vi "Test_PublishDblX_ObserveDblX_ValueReceived.vi"(8 "error in (no error)":errorcluster, 11 "TestCase in":refnum<class "TestModelPublishAndObserve.lvclass">) -> (0 "error out":errorcluster, 3 "TestCase out":refnum<class "TestModelPublishAndObserve.lvclass">)   [LabVIEW 2020, in "TestModelPublishAndObserve.lvclass"]
uses:
  TestModelPublishAndObserve.lvclass
  TestModelPublishAndObserve.lvclass/TestModelPublishAndObserve.ctl
  24bf8875-c008-4f22-9bfa-88e42476d167.vi
  Source/IModel/IModel/IModel.lvclass
  Doubles/RootModelPublishesDoubleFloatX/RootModelPublishesDoubleFloatX.lvclass
  C:/Git/mva-core/Source/RootModel/RootModel/RootModel.lvclass
  C:/Git/mva-core/Source/IModel/IModel/IModel.lvclass
  C:/Git/mva-core/Source/IObserver/IObserver/IObserver.lvclass
  C:/Program Files (x86)/National Instruments/LabVIEW 2020/vi.lib/ActorFramework/Actor/Actor.lvclass
  C:/Git/mva-core/Test/Doubles/RootModelPublishesDoubleFloatX/RootModelPublishesDoubleFloatX.lvclass
  <vilib>/ActorFramework/Actor/Actor.lvclass
  Source/Mediator/Mediator/Mediator.lvclass
  Doubles/ModelSubscribesToDoubleFloatX/ModelSubscribesToDoubleFloatX.lvclass
  <vilib>/ActorFramework/Stop Msg/Stop Msg.lvclass
  C:/Git/mva-core/Test/Doubles/ModelSubscribesToDoubleFloatX/ModelSubscribesToDoubleFloatX.lvclass
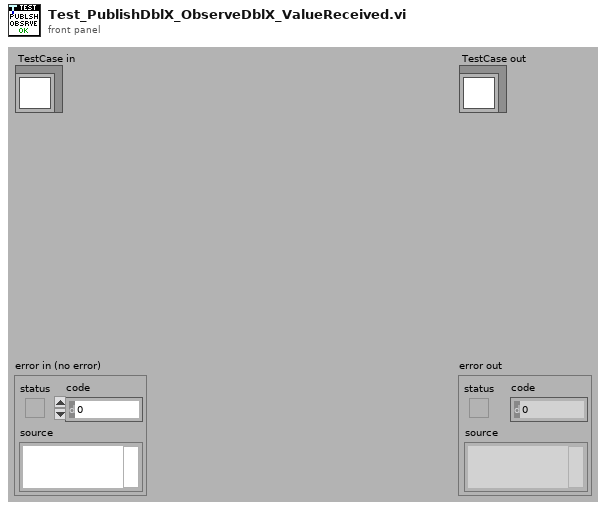
[diagram p1: front panel]
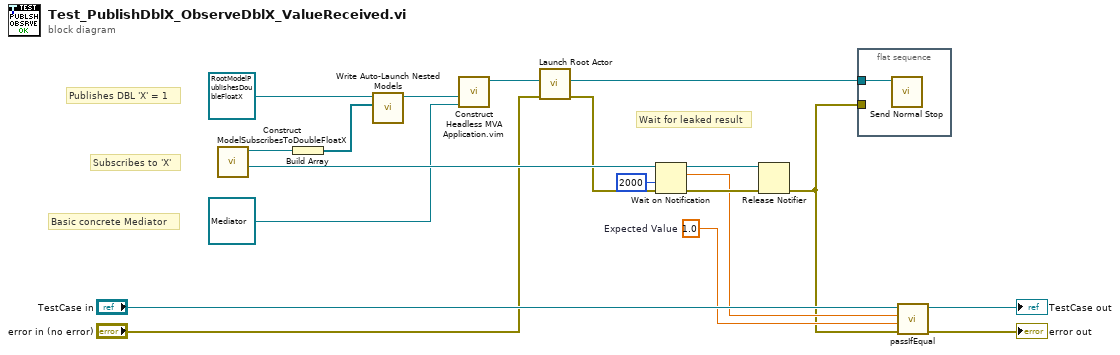
[diagram p0: block diagram]
diagram:
  w4 = 1.0  # Expected Value
  # "Wait for leaked result"
  # "Basic concrete Mediator"
  # "Subscribes to 'X'"
  # "Publishes DBL 'X' = 1"
  n1 = call "Construct ModelSubscribesToDoubleFloatX.vi"() -> ("Test Result Notifier"=w11:refnum<notifier>, "ModelSubscribesToDoubleFloatX"=w12:refnum<class "ModelSubscribesToDoubleFloatX.lvclass">)  [unwired: 10 in]
  n2 = Build Array(w12) -> (w15:refnum<class "ModelSubscribesToDoubleFloatX.lvclass">[])
  n3 = call "Write Auto-Launch Nested Models.vi"("Auto-Launch Nested Models"=w15, "IModel In"=refnum<class "RootModelPublishesDoubleFloatX.lvclass"> refnum ("RootModelPublishesDoubleFloatX.lvclass")) -> ("IModel Out"=w14:refnum<class "RootModelPublishesDoubleFloatX.lvclass">)  [unwired: 9 in]
  n4 = call "Construct Headless MVA Application.vim"("Mediator Type"=refnum<class "Mediator.lvclass"> refnum ("Mediator.lvlib:Mediator.lvclass"), "RootModel in"=w14) -> ("RootModel out"=w13:refnum<class "RootModelPublishesDoubleFloatX.lvclass">)  [unwired: 9 in]
  n5 = call <vilib>:"Launch Root Actor.vi"("error in (no error)"="error in (no error)", "Actor"=w13) -> ("error out"=w6:errorcluster, "Actor's Enqueuer"=w3:refnum<class "Message Enqueuer.lvclass">)  [unwired: 8 in]
  n6 = Wait on Notification(notifier=w11, timeout in ms (-1)=2000, error in (no error)=w6) -> (notifier out=w10:refnum<notifier>, notification=w5:dbl, error out=w8:errorcluster)  [unwired: 1 in, 1 out]
  n7 = Release Notifier(notifier=w10, error in (no error)=w8) -> (error out=w2:errorcluster)  [unwired: 1 in, 2 out]
  n8 = flat-sequence {
    tunnel: w3 -> [w20]
    tunnel: w2 -> [_]
    frame #0 {
      n9 = call <vilib>:"Send Normal Stop.vi"("Message Enqueuer"=w20) -> ()  [unwired: 10 in, 1 out]
    }
  }
  n10 = call-dynamic "passIfEqual.vi"("error in (no error)"=w2, "y"=w4, "x"=w5, "TestCase in"="TestCase in") -> ("error out"=→"error out":errorcluster, "TestCase out"=→"TestCase out":refnum<class "TestModelPublishAndObserve.lvclass">)  [unwired: 6 in]
